vi "KILL.vi"() -> ()   [LabVIEW 2020]
panel:
  in  "Nom de ressource VISA":refnum<visa-resource-name>
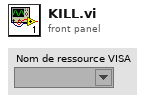
[diagram p1: front panel]
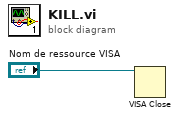
[diagram p0: block diagram]
diagram:
  n1 = VISA Close(VISA resource name="Nom de ressource VISA") -> ()  [unwired: 1 in, 1 out]
